vi "Execute.vi"(8 "error in (no error)":errorcluster, 10 "Context in":refnum<class "Context.lvclass">, 11 "Manual Mode Command In":refnum<class "Manual Mode Command.lvclass">) -> (0 "error out":errorcluster, 2 "Context out":refnum<class "Context.lvclass">, 3 "Manual Mode Command out":refnum<class "Manual Mode Command.lvclass">)   [LabVIEW 2016, in "Manual Mode Command.lvclass"]
uses:
  Manual Mode Command.lvclass
  Context/Context.lvclass
  Manual Mode Command.lvclass/Manual Mode Command.ctl
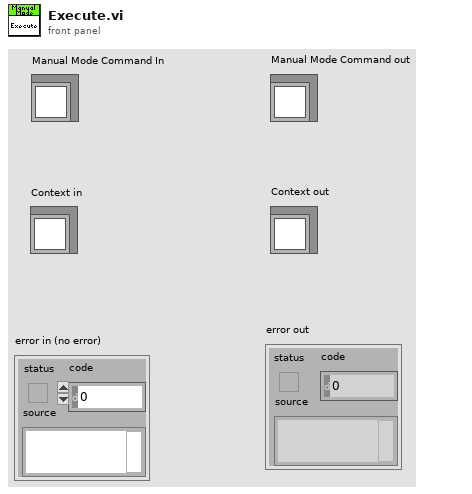
[diagram p1: front panel]
types:
  T1 = typedef "HPMT_Typedefs.lvlib/TestSettings.ctl" = cluster{"Operator":string, "Strut Number":string, "Test Stand Serial Number":string, "Notes":string, "Test Angle":u16, "Number of Cycles":u16, "Data Points per Cycle":u16, "Settling Time (secs)":u16, "Breakaway Air Pressure":u16, "Largest Strut Displacement":dbl}
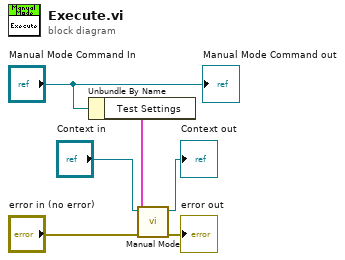
[diagram p0: block diagram]
diagram:
  n1 = Unbundle By Name("Manual Mode Command In") -> ("Test Settings"=w1:T1)
  n2 = call "Manual Mode.vi"("error in (no error)"="error in (no error)", "Test Settings"=w1, "Context in"="Context in") -> ("error out"=→"error out":errorcluster, "Context out"=→"Context out":refnum<class "Context.lvclass">)  [unwired: 7 in]
  "Manual Mode Command out" <- "Manual Mode Command In"
